vi "Node.Settings.vi"(6 "Action":enum8{"Get", "Set"}(ring), 8 "error in (no error)":errorcluster, 10 "Node.Settings":T1 {"Name" format="%.0x"}, 11 "Item Ref in":T2 format="%.0x") -> (0 "error out":errorcluster, 2 "Node.Settings":T1 {"Name" format="%.0x"}, 3 "Item Ref out":T2 format="%.0x")   [LabVIEW 2015, in "J1939 Addon System Explorer.lvlib"]
uses:
  J1939 Addon System Explorer.lvlib
  <vilib>/NI Veristand/Custom Device API/Custom Device Item Ref.ctl
  Shared/Types/Monitor Settings.ctl
  Shared/SubVIs/Constants.vi
  <vilib>/NI/NIVS System Definition Utilities/_SubVIs/SysDef.Property.Set.U32.vi
  <vilib>/NI/NIVS System Definition Utilities/_SubVIs/SysDef.Property.Set.String.vi
  <vilib>/NI Veristand/Custom Device API/Get Item Property (U32).vi
  <vilib>/NI Veristand/Custom Device API/Get Item Property (String).vi
  <vilib>/NI VeriStand/Custom Device API/Custom Device API.lvlib
  Shared/J1939 Addon Shared.lvlib
  <vilib>/NI/NIVS System Definition Utilities/System Definition Utilities.lvlib
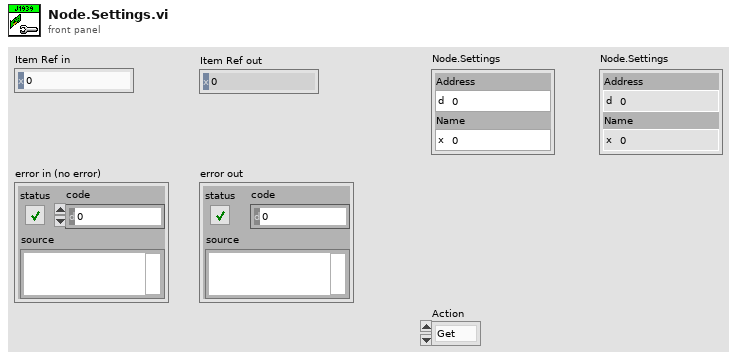
[diagram p1: front panel]
types:
  T1 = typedef "J1939 Addon Shared.lvlib/Monitor Settings.ctl" = cluster{"Address":u8, "Name":u64}
  T2 = typedef "Custom Device API.lvlib/Custom Device Item Ref.ctl" = u64
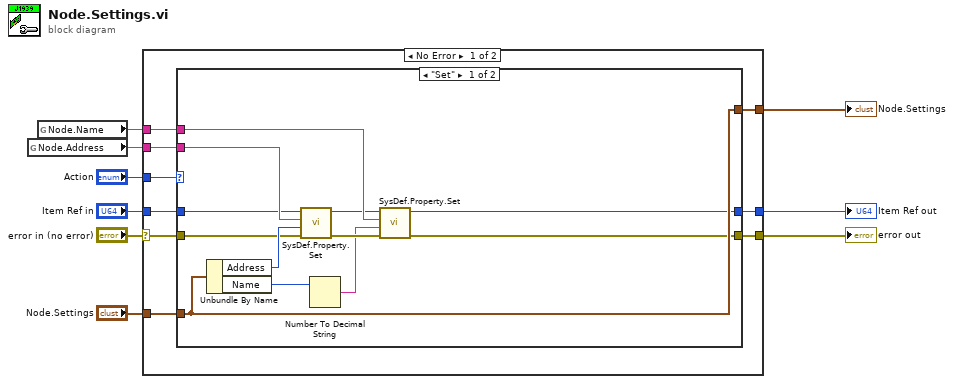
[diagram p0: block diagram]
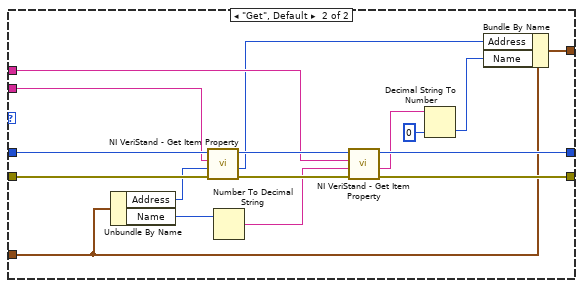
[diagram p2: hidden frame]
diagram:
  n1 = global read "Constants.vi" "Node.Address"() -> (w8:string)
  n2 = global read "Constants.vi" "Node.Name"() -> (w4:string)
  n3 = case shown="No Error" "error in (no error)" {
    selector: "error in (no error)" -> [w12 w49]
    tunnel: "Item Ref in" -> [w18 w48]
    tunnel: w8 -> [w17 _]
    tunnel: [w16 w49] -> w7
    tunnel: [w15 w48] -> w6
    tunnel: [w14 _] -> w5
    tunnel: w4 -> [w13 _]
    tunnel: "Node.Settings" -> [w11 _]
    tunnel: "Action" -> [w10 _]
    frame No Error {
      n4 = case shown="\"Set\"" w10 {
        tunnel: w18 -> [w27 w41]
        tunnel: w17 -> [w30 w37]
        tunnel: [w21 w44] -> w16
        tunnel: [w20 w43] -> w15
        tunnel: [w28 w47] -> w14
        tunnel: w13 -> [w29 w36]
        tunnel: w12 -> [w22 w42]
        tunnel: w11 -> [w28 w39]
        frame "Set" {
          n5 = Unbundle By Name(w28) -> ("Address"=w24:u8, "Name"=w23:u64)
          n6 = call-poly <vilib>:"SysDef.Property.Set.vi"("error in (no error)"=w22, "Value"=w24, "Property Name"=w30, "nodeID"=w27) -> ("error out"=w26:errorcluster, "nodeID out"=w25:u64)  [unwired: 6 in]
          n7 = Number To Decimal String(number=w23) -> (decimal integer string=w19:string)  [unwired: 1 in]
          n8 = call-poly <vilib>:"SysDef.Property.Set.vi"("error in (no error)"=w26, "Value"=w19, "Property Name"=w29, "nodeID"=w25) -> ("error out"=w21:errorcluster, "nodeID out"=w20:u64)  [unwired: 6 in]
        }
        frame "Get", Default {
          n9 = Unbundle By Name(w39) -> ("Address"=w38:u8, "Name"=w40:u64)
          n10 = call-poly <vilib>:"NI VeriStand - Get Item Property.vi"("error in (no error)"=w42, "Default Value"=w38, "Property Name"=w37, "Item Ref in"=w41) -> ("error out"=w46:errorcluster, "Value"=w34:u32, "Item Ref out"=w45:T2)  [unwired: 4 in, 1 out]
          n11 = Number To Decimal String(number=w40) -> (decimal integer string=w35:string)  [unwired: 1 in]
          n12 = call-poly <vilib>:"NI VeriStand - Get Item Property.vi"("error in (no error)"=w46, "Default Value"=w35, "Property Name"=w36, "Item Ref in"=w45) -> ("error out"=w44:errorcluster, "Value"=w33:string, "Item Ref out"=w43:T2)  [unwired: 4 in, 1 out]
          n13 = Decimal String To Number(string=w33, default (0L)=u64 0 ("default (0 I32)")) -> (number=w31:u64)  [unwired: 1 in, 1 out]
          n14 = Bundle By Name(cluster=w39, "Address"=w34, "Name"=w31) -> (w47:T1)
        }
      }
    }
    frame Error {
    }
  }
  "Item Ref out" <- w6
  "error out" <- w7
  "Node.Settings" <- w5
